vi "ConfigureTrigger.vi"(8 "error in (no error)":errorcluster, 11 "SpecAnBase in":refnum<class "SpecAnBase.lvclass">) -> (0 "error out":errorcluster, 3 "SpecAnBase out":refnum<class "SpecAnBase.lvclass">)   [LabVIEW 2018, in "SpecAnPlugins.lvlib" / "SpecAnBase.lvclass"]
doc: "This function allows the user to configuree the Spectrum Analyser to acquire measurements based on a software, external, video or etc signal and the associated paramater such as level and slope."
uses:
  SpecAnBase.lvclass
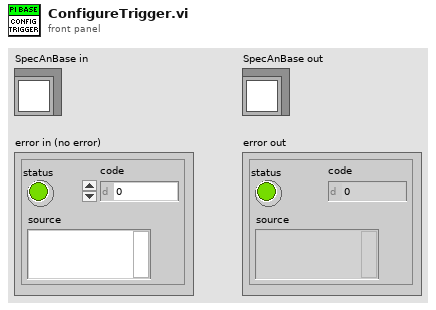
[diagram p1: front panel]
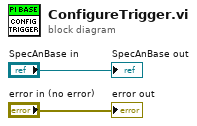
[diagram p0: block diagram]
diagram:
  "error out" <- "error in (no error)"
  "SpecAnBase out" <- "SpecAnBase in"
